vi "RSZVB Set Mixer Constant Delay Enabled.vi"(8 "error in (no error)":errorcluster {"code" format="%.0x"}, 9 "Constant Delay (Off)":bool, 10 "Channel (1)":i32=1, 11 "VISA session":refnum<visa-resource-name>) -> (0 "error out":errorcluster {"code" format="%.0x"}, 3 "dup VISA session":refnum<visa-resource-name>)   [LabVIEW 2011]
doc: "Selects constant or variable delay for the mixer delay calibration.\n\nRemote-control command(s):\n[SENSe<Ch>:]FREQuency:MDELay:CDMode ON|OFF"
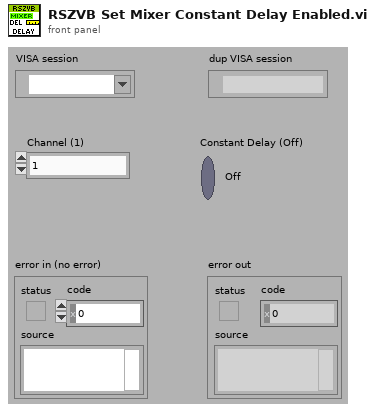
[diagram p1: front panel]
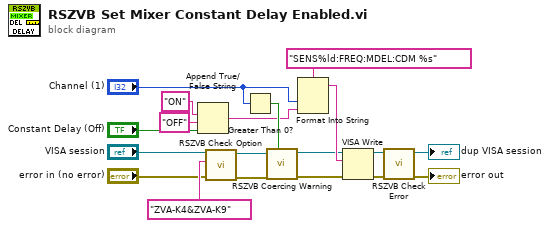
[diagram p0: block diagram]
diagram:
  n1 = Append True/False String(1:"Constant Delay (Off)", 2:"OFF" ("false string"), 3:"ON" ("true string")) -> (0:w10:string)  [unwired: 1 in]
  n2 = call "RSZVB Check Option.vi"("error in (no error)"="error in (no error)", "Options"="ZVA-K4&ZVA-K9", "VISA session"="VISA session") -> ("error out"=w1:errorcluster, "dup VISA session"=w2:refnum<visa-resource-name>)  [unwired: 7 in]
  n3 = Greater Than 0?(x="Channel (1)") -> (x > 0?=w11:bool)
  n4 = call "RSZVB Coercing Warning.vi"("In Range?"=w11, "error in (no error)"=w1, "VISA session"=w2) -> ("error out"=w16:errorcluster, "dup VISA session"=w15:refnum<visa-resource-name>)  [unwired: 7 in]
  n5 = Format Into String(format string="SENS%ld:FREQ:MDEL:CDM %s", "Channel (1)", w10) -> (resulting string=w19:string)  [unwired: 2 in, 1 out]
  n6 = VISA Write(VISA resource name=w15, write buffer=w19, error in (no error)=w16) -> (VISA resource name out=w18:refnum<visa-resource-name>, error out=w17:errorcluster)  [unwired: 1 out]
  n7 = call "RSZVB Check Error.vi"("error in (no error)"=w17, "VISA session"=w18) -> ("error out"=→"error out":errorcluster, "dup VISA session"=→"dup VISA session":refnum<visa-resource-name>)  [unwired: 8 in]
